vi "Build string table.vi"(1 "row headers":string[](array[string]), 2 "column headers":string[](array[string]), 3 "text data":string[][](array[string])) -> (0 "output table":string[][](array[string]))   [LabVIEW 2020, in "NI_ReportGenerationToolkit.lvlib"]
uses:
  <vilib>/addons/_office/NI_ReportGenerationToolkit.lvlib
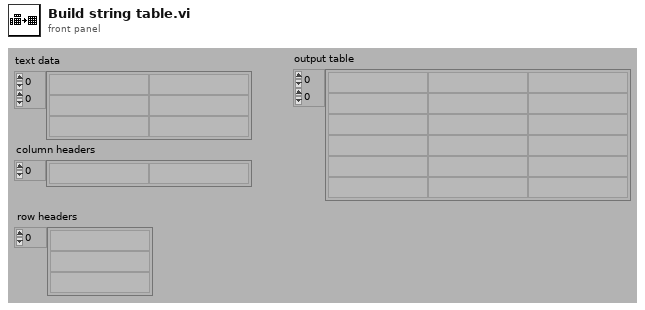
[diagram p1: front panel]
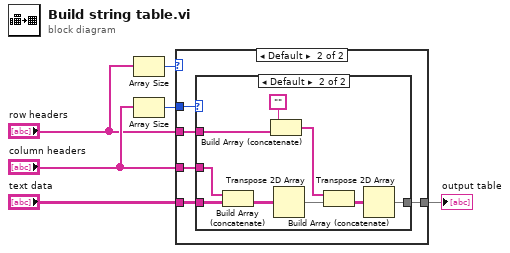
[diagram p0: block diagram]
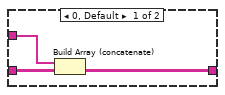
[diagram p3: hidden frame]
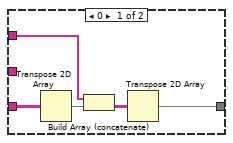
[diagram p4: hidden frame]
diagram:
  n1 = Array Size(array="row headers") -> (size(s)=w2:i32)
  n2 = Array Size(array="column headers") -> (size(s)=w1:i32)
  n3 = case shown="Default" w2 {
    tunnel: [w7 w19] -> w6
    tunnel: "column headers" -> [w9 w18]
    tunnel: w1 -> [w10 w17]
    tunnel: "text data" -> [w8 w16]
    tunnel: "row headers" -> [_ w15]
    frame 0 {
      n4 = case shown="1" w10 {
        tunnel: w9 -> [w13 _]
        tunnel: w8 -> [w12 w14]
        tunnel: [w11 w14] -> w7
        frame 0, Default {
          n5 = Build Array (concatenate)(w13, w12) -> (w11:string[][])
        }
        frame 1 {
          # "no row or column headers"
        }
      }
    }
    frame Default {
      n6 = case shown="Default" w17 {
        tunnel: [w21 w31] -> w19
        tunnel: w18 -> [_ w28]
        tunnel: w16 -> [w23 w27]
        tunnel: w15 -> [w24 w25]
        frame 0 {
          n7 = Transpose 2D Array(2D array=w23) -> (transposed array=w22:string[][])
          n8 = Build Array (concatenate)(w24, w22) -> (w20:string[][])
          n9 = Transpose 2D Array(2D array=w20) -> (transposed array=w21:string[][])
        }
        frame Default {
          n10 = Build Array (concatenate)(w28, w27) -> (w26:string[][])
          n11 = Build Array (concatenate)("", w25) -> (w29:string[])
          n12 = Transpose 2D Array(2D array=w26) -> (transposed array=w30:string[][])
          n13 = Build Array (concatenate)(w29, w30) -> (w32:string[][])
          n14 = Transpose 2D Array(2D array=w32) -> (transposed array=w31:string[][])
        }
      }
    }
  }
  "output table" <- w6
